vi "Sonar safety.vi"(0 "M1 input":dbl format="%#_4g", 1 "M2 input":dbl format="%#_4g") -> (2 "M1 Output":dbl format="%#_4g", 4 "M2 output":dbl format="%#_4g")   [LabVIEW 2012]
doc: "This example shows how to use the MaxBotix LV-MaxSonar-EZ1 Sonar Range Finder MB1010. It will display the distance from the sensor in inches.\n\nThis example works with the NI 9403 module connected to a Digital Sidecar. The Digital Sidecar should have 12V applied to the WAGO connector. The sensor is attached to the 3x8 header using a 3-pin PWM connector."
uses:
  Robot Global Data.vi
panel:
  out "distance rear":dbl(slide)=125.0 scale=0.0..250.0 scale format="%3d"
  out "distance front":dbl(slide)=125.0 scale=0.0..250.0 scale format="%3d"
  # "Output information."
  # "EZ1"
  # "inches"
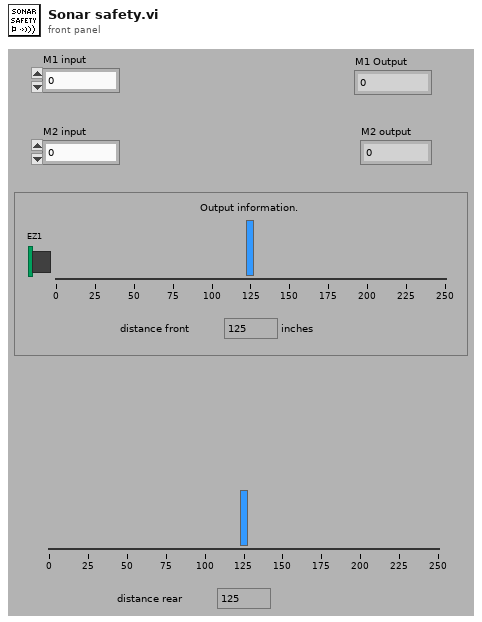
[diagram p1: front panel]
types:
  T1 = typedef "WPI_CounterDevRef.ctl" = cluster{"DevStatus":errorcluster, "CntIndex":T2}
  T2 = typedef "FPGA_CounterCtrSystemIndex.ctl" = enum8{"Ctr 0", "Ctr 1", "Ctr 2", "Ctr 3", "Ctr 4", "Ctr 5", "Ctr 6", "Ctr 7", "Invalid"}
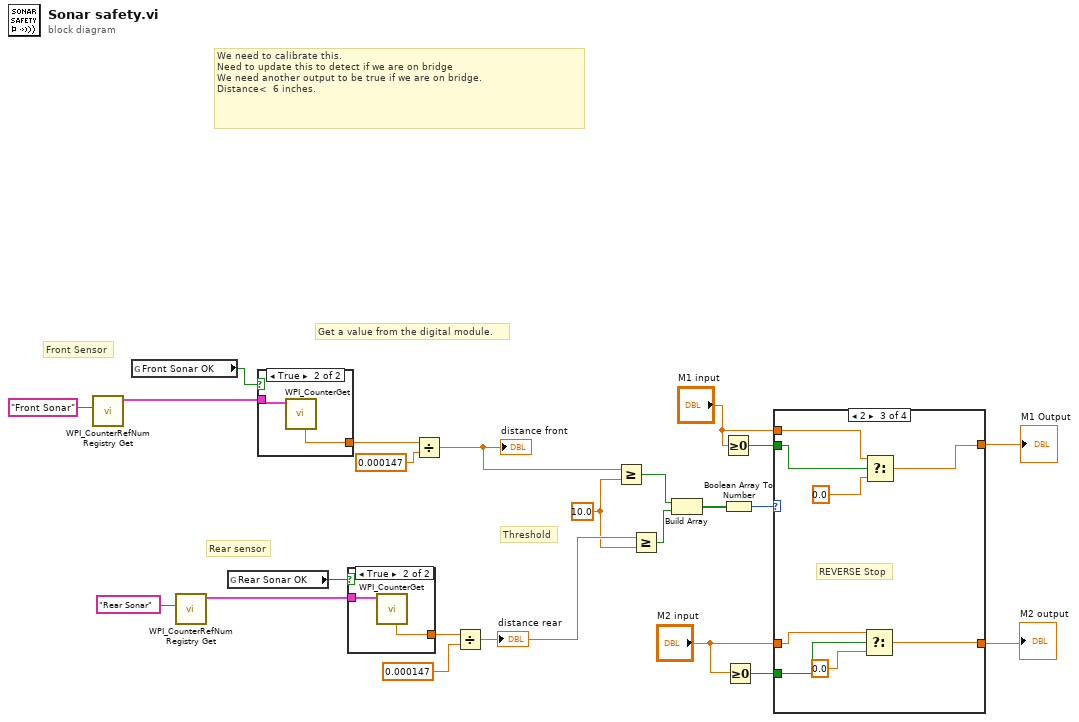
[diagram p0: block diagram]
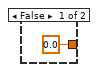
[diagram p2: hidden frame]
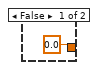
[diagram p3: hidden frame]
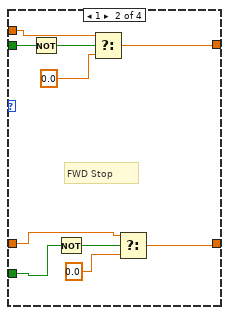
[diagram p5: hidden frame]
diagram:
  w20 = 10.0 ("y")
  # "Rear sensor"
  # "Front Sensor"
  # "Threshold"
  # "We need to calibrate this.\nNeed to update this to detect if we are on bridge\nWe need another output to be true if we are on bridge.\nDistance<  6 inches."
  # "Get a value from the digital module."
  n1 = call <vilib>:"WPI_CounterRefNum Registry Get.vi"("refnum name"="Front Sonar") -> ("CounterDevRef"=w5:T1)  [unwired: 9 in, 1 out]
  n2 = global read "Robot Global Data.vi" "Front Sonar OK"() -> (w2:bool)
  n3 = call <vilib>:"WPI_CounterRefNum Registry Get.vi"("refnum name"="Rear Sonar") -> ("CounterDevRef"=w4:T1)  [unwired: 9 in, 1 out]
  n4 = global read "Robot Global Data.vi" "Rear Sonar OK"() -> (w1:bool)
  n5 = case shown="True" w2 {
    tunnel: [0.0 ("Period (sec)") w26] -> w8
    tunnel: w5 -> [_ w25]
    frame False {
    }
    frame True {
      n6 = call <vilib>:"WPI_CounterGet.vi"("CounterDevRef in"=w25) -> ("Period (sec)"=w26:dbl)  [unwired: 5 in, 5 out]
    }
  }
  n7 = case shown="True" w1 {
    tunnel: [0.0 ("Period (sec)") w29] -> w3
    tunnel: w4 -> [_ w28]
    frame False {
    }
    frame True {
      n8 = call <vilib>:"WPI_CounterGet.vi"("CounterDevRef in"=w28) -> ("Period (sec)"=w29:dbl)  [unwired: 5 in, 5 out]
    }
  }
  n9 = Divide(x=w8, y=0.000147 ("Scaling factor (s/in)")) -> (x/y=w22:dbl)
  "distance front" <- w22
  n10 = Divide(x=w3, y=0.000147 ("Scaling factor (s/in)")) -> (x/y=w21:dbl)
  "distance rear" <- w21
  n11 = Greater Or Equal?(x=w22, y=w20) -> (x >= y?=w16:bool)
  n12 = Greater Or Equal?(x=w21, y=w20) -> (x >= y?=w15:bool)
  n13 = Build Array(w16, w15) -> (w14:bool[])
  n14 = Greater Or Equal To 0?(x="M1 input") -> (x >= 0?=w11:bool)
  n15 = Boolean Array To Number(Boolean array=w14) -> (number=w13:u32)
  n16 = Greater Or Equal To 0?(x="M2 input") -> (x >= 0?=w9:bool)
  n17 = case shown="2" w13 {
    tunnel: "M1 input" -> [w31 w38 w43 w51]
    tunnel: [w31 w40 w42 w51] -> w19
    tunnel: w11 -> [_ w39 w44 _]
    tunnel: "M2 input" -> [w30 w32 w46 w50]
    tunnel: [w30 w33 w45 w50] -> w18
    tunnel: w9 -> [_ w34 w47 _]
    frame 0, Default {
      # "Both sensors are OK"
    }
    frame 1 {
      # "FWD Stop"
      n18 = Not(x=w39) -> (.not. x?=w37:bool)
      n19 = Not(x=w34) -> (.not. x?=w36:bool)
      n20 = Select(t=w38, s=w37, f=0.0) -> (s? t:f=w40:dbl)
      n21 = Select(t=w32, s=w36, f=0.0) -> (s? t:f=w33:dbl)
    }
    frame 2 {
      # "REVERSE Stop"
      n22 = Select(t=w46, s=w47, f=0.0) -> (s? t:f=w45:dbl)
      n23 = Select(t=w43, s=w44, f=0.0) -> (s? t:f=w42:dbl)
    }
    frame 3 {
      # "Probably fell\nOver or no sensors\nWorking"
    }
  }
  "M1 Output" <- w19
  "M2 output" <- w18
